vi "Acquire.vi"(8 "error in (no error)":errorcluster, 10 "Msg in":T1, 11 "FakePressureController in":refnum<class "Tapedrive_ESP301.lvclass">) -> (0 "error out":errorcluster, 1 "new command":string, 2 "Msg out":T1, 3 "FakePressureController out":refnum<class "Tapedrive_ESP301.lvclass">)   [LabVIEW 2013, in "Tapedrive_ESP301.lvclass"]
uses:
  Tapedrive_ESP301.lvclass
  BaseDriver/BaseDriver.lvclass
  shared/OnOffTypeDef.ctl
  shared/CompressAndUpdate(Poly)/CompressAndUpdate(Enum).vi
  shared/CompressAndUpdate(Poly)/CompressAndUpdate(Numeric).vi
  BaseDriver/DriverMsg.ctl
panel:
  out "moving 2":bool
  out "moving 1":bool
  out "x .or. y?":bool
  out "Error Code":i32[](array[numeric])
  out "Error Message":string
  out "x-y":u32(graph)
  out "result":bool
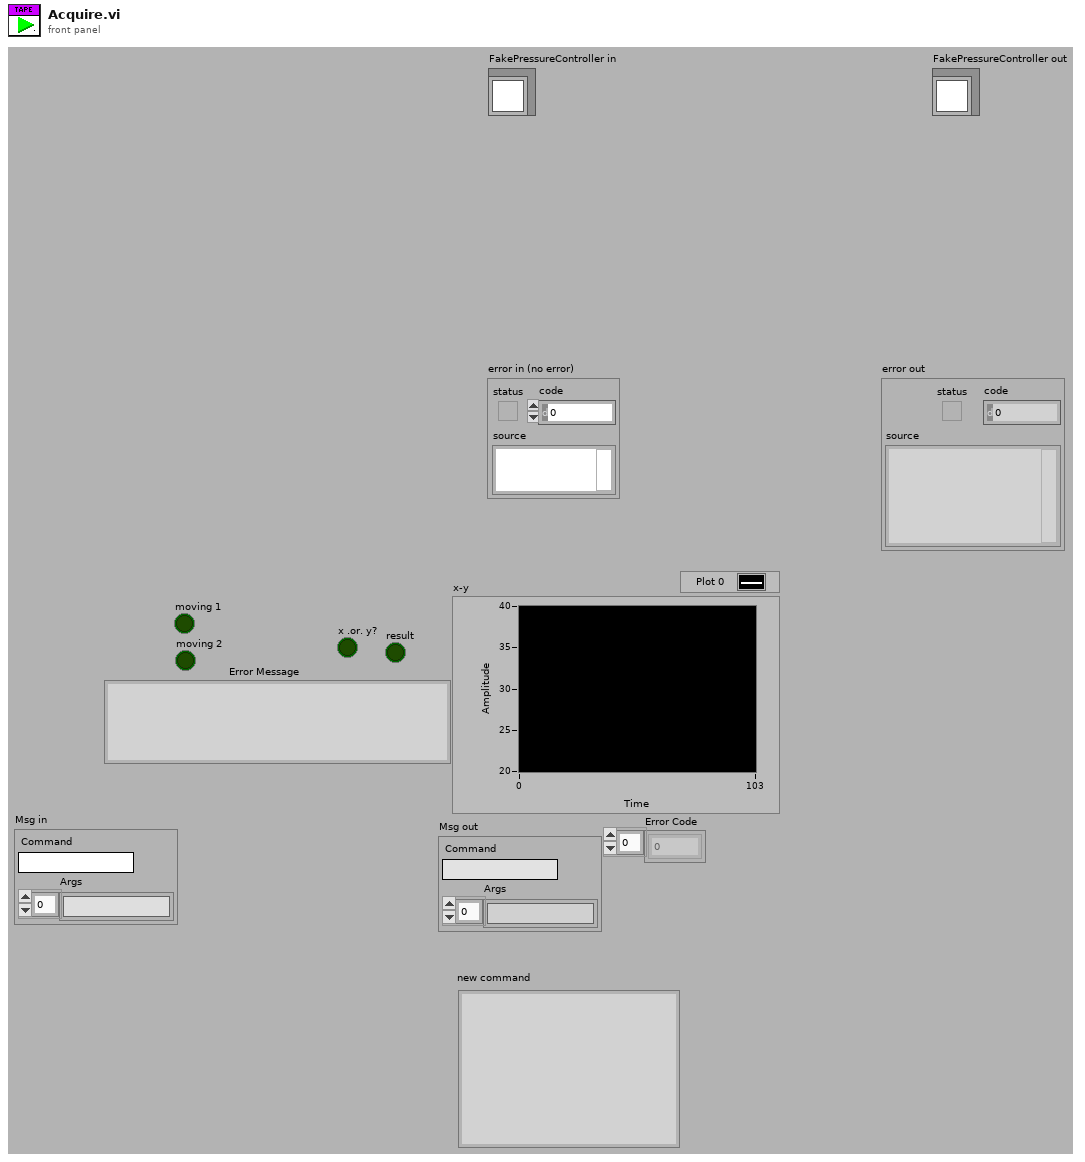
[diagram p1: front panel]
types:
  T1 = typedef "DriverMsg.ctl" = cluster{"Command":string, "Args":string[]}
  T2 = typedef "OnOffTypeDef.ctl" = enum16{"off", "on"}
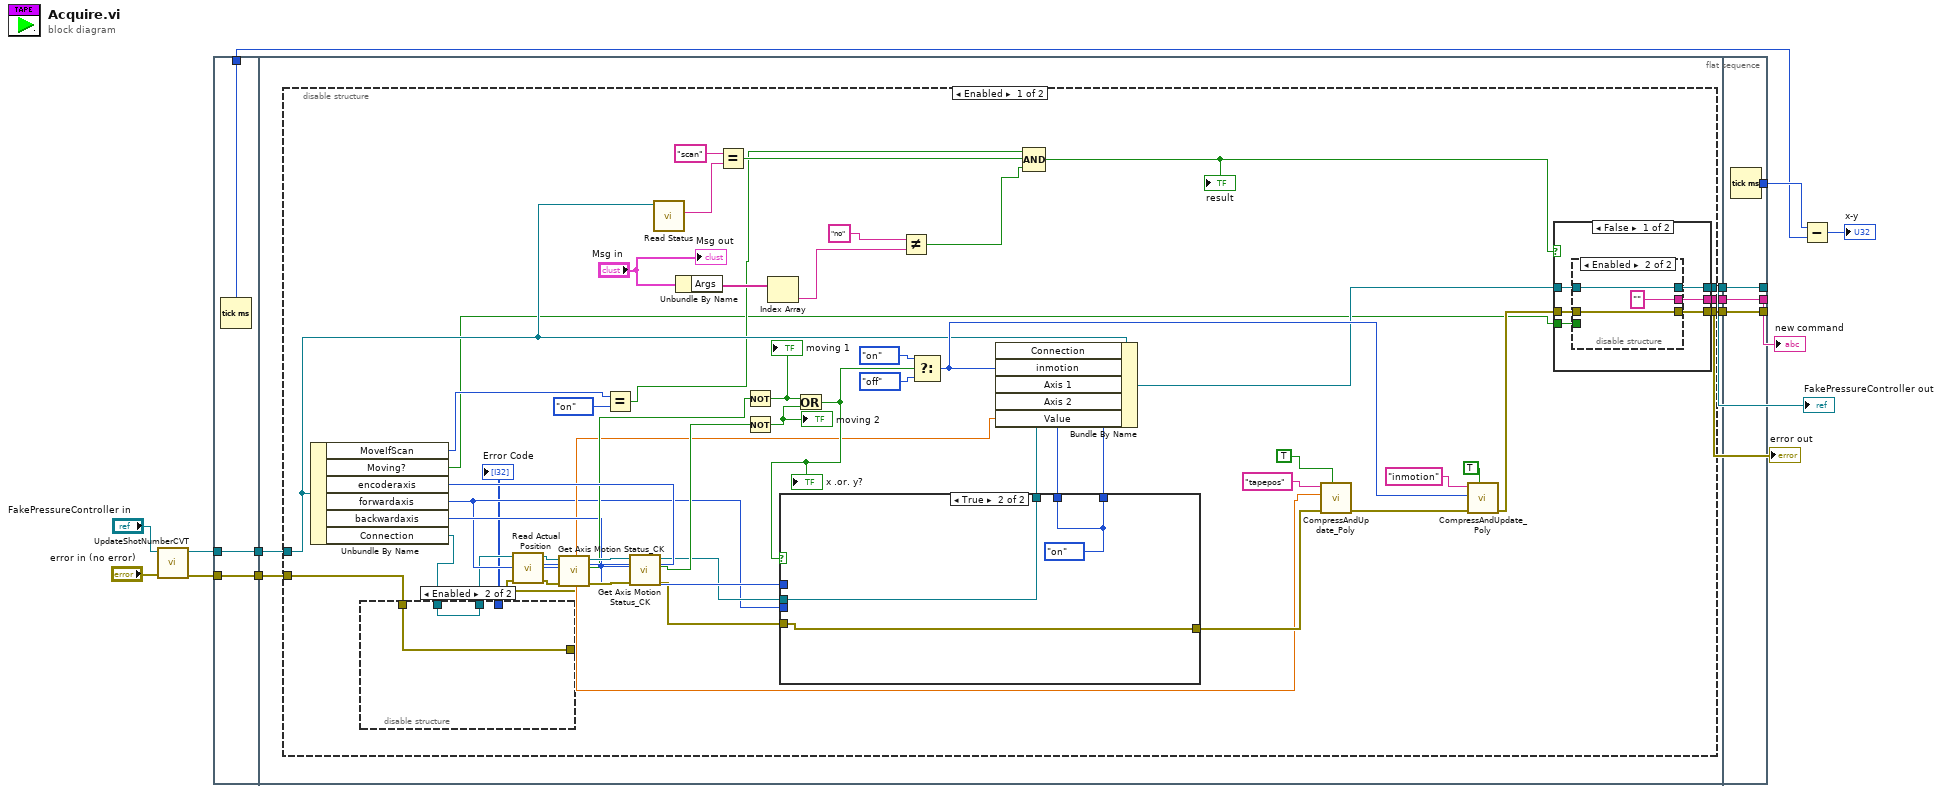
[diagram p0: block diagram]
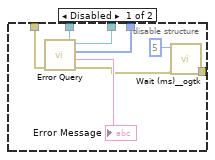
[diagram p2: hidden frame]
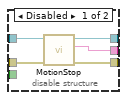
[diagram p3: hidden frame]
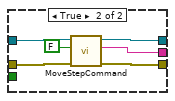
[diagram p4: hidden frame]
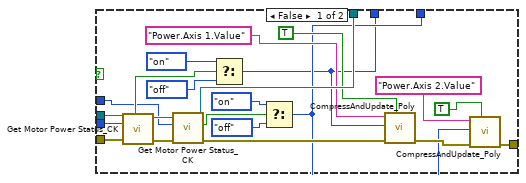
[diagram p5: hidden frame]
diagram:
  n1 = call "UpdateShotNumberCVT.vi"("error in (no error)"="error in (no error)", "BaseDriver in"="FakePressureController in") -> ("error out"=w9:errorcluster, "BaseDriver out"=w11:refnum<class "Tapedrive_ESP301.lvclass">)  [unwired: 8 in]
  n2 = flat-sequence {
    tunnel: w9 -> [w17]
    tunnel: w11 -> [w18]
    tunnel: [w18] -> w5
    tunnel: [w17] -> w4
    tunnel: [w16] -> w2
    tunnel: [w23] -> w8
    tunnel: [w22] -> w7
    tunnel: [w20] -> w6
    tunnel: w5 -> [w21]
    tunnel: w4 -> [w19]
    tunnel: [w133] -> w10
    tunnel: [w134] -> w12
    tunnel: [w135] -> w13
    tunnel: w8 -> [w135]
    tunnel: w7 -> [w134]
    tunnel: w6 -> [w133]
    tunnel: [w132] -> w3
    frame #0 {
      n3 = Tick Count (ms)() -> (millisecond timer value=w16:u32)
    }
    frame #1 {
      n4 = disable-structure shown="Enabled" {
        disable-tunnel: [w53 w130] -> w23
        disable-tunnel: [w52 w131] -> w22
        disable-tunnel: w21 -> [w51 w131]
        disable-tunnel: [w44 _] -> w20
        disable-tunnel: w19 -> [w27 w130]
        frame Enabled {
          n5 = Unbundle By Name(w51) -> ("MoveIfScan"=w39:T2, "Moving?"=w34:bool, "encoderaxis"=w70:i16, "forwardaxis"=w31:i16, "backwardaxis"=w60:i16, "Connection"=w29:refnum<visa-resource-name>)
          n6 = disable-structure shown="Enabled" {
            disable-tunnel: w29 -> [w82 w84]
            disable-tunnel: [w81 w84] -> w28
            disable-tunnel: w27 -> [w80 w83]
            disable-tunnel: [w78 _] -> w26
            disable-tunnel: [w76 w83] -> w25
            frame Disabled {
              n7 = call <instrlib>:"Error Query.vi"("error in (no error)"=w80, "VISA resource name"=w82) -> ("error out"=w77:errorcluster, "Error Message"=→"Error Message":string, "Error Code"=w78:i32[], "VISA resource name out"=w81:refnum<visa-resource-name>)  [unwired: 2 out]
              n8 = call <userlib>:"Wait (ms)__ogtk.vi"("error in (no error)"=w77, "milliseconds to wait"=u32 5) -> ("error out"=w76:errorcluster)  [unwired: 8 in, 1 out]
            }
            frame Enabled {
            }
          }
          "Error Code" <- w26
          n9 = call <instrlib>:"Read Actual Position.vi"("error in (no error)"=w25, "Axis (1)"=w70, "VISA resource name"=w28) -> ("error out"=w30:errorcluster, "Position (units)"=w33:dbl, "VISA resource name out"=w32:refnum<visa-resource-name>)  [unwired: 2 in]
          n10 = call "Get Axis Motion Status_CK.vi"("error in (no error)"=w30, "Axis (1)"=w31, "VISA resource name"=w32) -> ("error out"=w72:errorcluster, "Motion Done"=w69:bool, "VISA resource name out"=w71:refnum<visa-resource-name>)  [unwired: 2 in]
          n11 = Equal?(x=w39, y=OnOffTypeDef."on") -> (x = y?=w37:bool)
          n12 = call "Get Axis Motion Status_CK.vi"("error in (no error)"=w72, "Axis (1)"=w60, "VISA resource name"=w71) -> ("error out"=w36:errorcluster, "Motion Done"=w68:bool, "VISA resource name out"=w35:refnum<visa-resource-name>)  [unwired: 2 in]
          n13 = call "Read Status.vi"("BaseDriver in"=w51) -> ("Status"=w40:string)  [unwired: 8 in, 2 out]
          n14 = Unbundle By Name("Msg in") -> ("Args"=w49:string[])
          n15 = Equal?(x="scan", y=w40) -> (x = y?=w41:bool)
          n16 = Not(x=w69) -> (.not. x?=w67:bool)
          "moving 1" <- w67
          n17 = Not(x=w68) -> (.not. x?=w24:bool)
          "moving 2" <- w24
          n18 = Index Array(array=w49) -> (element=w48:string)  [unwired: 1 in]
          n19 = Or(x=w67, y=w24) -> (x .or. y?=w43:bool)
          "x .or. y?" <- w43
          n20 = case shown="True" w43 {
            tunnel: w36 -> [w126 w127]
            tunnel: w35 -> [w124 w129]
            tunnel: [w122 w129] -> w61
            tunnel: w31 -> [w115 _]
            tunnel: w60 -> [w114 _]
            tunnel: [w107 w127] -> w59
            tunnel: [w106 w128] -> w57
            tunnel: [w105 w128] -> w56
            frame False {
              n21 = call "Get Motor Power Status_CK.vi"("error in (no error)"=w126, "Axis (1)"=w115, "VISA resource name"=w124) -> ("error out"=w125:errorcluster, "Power Status"=w117:bool, "VISA resource name out"=w123:refnum<visa-resource-name>)  [unwired: 2 in]
              n22 = call "Get Motor Power Status_CK.vi"("error in (no error)"=w125, "Axis (1)"=w114, "VISA resource name"=w123) -> ("error out"=w109:errorcluster, "Power Status"=w116:bool, "VISA resource name out"=w122:refnum<visa-resource-name>)  [unwired: 2 in]
              n23 = Select(t=OnOffTypeDef."on" ("Settings.inmotion"), s=w117, f=OnOffTypeDef."off" ("Settings.inmotion")) -> (s? t:f=w105:T2)
              n24 = Select(t=OnOffTypeDef."on" ("Settings.inmotion"), s=w116, f=OnOffTypeDef."off" ("Settings.inmotion")) -> (s? t:f=w106:T2)
              n25 = call-poly "CompressAndUpdate_Poly.vi"("force CVT update (false)"=TRUE, "error in"=w109, "enum variant"=w105, "command or variable name"="Power.Axis 1.Value") -> ("error out"=w108:errorcluster)  [unwired: 7 in]
              n26 = call-poly "CompressAndUpdate_Poly.vi"("force CVT update (false)"=TRUE, "error in"=w108, "enum variant"=w106, "command or variable name"="Power.Axis 2.Value") -> ("error out"=w107:errorcluster)  [unwired: 7 in]
            }
            frame True {
              w128 = OnOffTypeDef."on" ("Settings.inmotion")
            }
          }
          n27 = Not Equal?(x="no", y=w48) -> (x != y?=w46:bool)
          n28 = Select(t=OnOffTypeDef."on" ("Settings.inmotion"), s=w43, f=OnOffTypeDef."off" ("Settings.inmotion")) -> (s? t:f=w58:T2)
          n29 = Bundle By Name(cluster=w51, "Connection"=w61, "inmotion"=w58, "Axis 1"=w56, "Axis 2"=w57, "Value"=w33) -> (w55:refnum<class "Tapedrive_ESP301.lvclass">)
          n30 = Compound Arithmetic op=AND(w37, w41, w46) -> (w45:bool)
          "result" <- w45
          n31 = call-poly "CompressAndUpdate_Poly.vi"("force CVT update (false)"=TRUE, "error in"=w59, "Numeric"=w33, "command or variable name"="tapepos") -> ("error out"=w63:errorcluster)  [unwired: 7 in]
          n32 = call-poly "CompressAndUpdate_Poly.vi"("force CVT update (false)"=TRUE, "error in"=w63, "enum variant"=w58, "command or variable name"="inmotion") -> ("error out"=w54:errorcluster)  [unwired: 7 in]
          n33 = case shown="False" w45 {
            tunnel: w55 -> [w90 w103]
            tunnel: w54 -> [w89 w101]
            tunnel: [w88 w100] -> w53
            tunnel: [w87 w102] -> w52
            tunnel: [w86 w104] -> w44
            tunnel: w34 -> [w85 _]
            frame False {
              n34 = disable-structure shown="Enabled" {
                disable-tunnel: w90 -> [w95 w97]
                disable-tunnel: w89 -> [w92 w96]
                disable-tunnel: [w93 w96] -> w88
                disable-tunnel: [w94 w97] -> w87
                disable-tunnel: [w91 "" ("new command")] -> w86
                disable-tunnel: w85 -> [_ _]
                frame Disabled {
                  n35 = call "MotionStop.vi"("error in (no error)"=w92, "Tapedrive_ESP301 in"=w95) -> ("error out"=w93:errorcluster, "new command"=w91:string, "Tapedrive_ESP301 out"=w94:refnum<class "Tapedrive_ESP301.lvclass">)  [unwired: 7 in]
                }
                frame Enabled {
                }
              }
            }
            frame True {
              n36 = call "MoveStepCommand.vi"("error in (no error)"=w101, "MultiCVT"=FALSE, "Tapedrive_ESP301 in"=w103) -> ("error out"=w100:errorcluster, "String"=w104:string, "Tapedrive_ESP301.lvclass"=w102:refnum<class "Tapedrive_ESP301.lvclass">)  [unwired: 6 in]
            }
          }
          "Msg out" <- "Msg in"
        }
        frame Disabled {
        }
      }
    }
    frame #2 {
      n37 = Tick Count (ms)() -> (millisecond timer value=w132:u32)
    }
  }
  n38 = Subtract(x=w3, y=w2) -> (x-y=→"x-y":u32)
  "error out" <- w13
  "FakePressureController out" <- w12
  "new command" <- w10
